vi "TS DotStar SPI V5 - Switched Style.vi"() -> ()   [LabVIEW 2016]
doc: "ADXL362 SPI Accelerometer\n\nThis example shows how to use the Analog Devices ADXL362 Accelerometer sensor connected to SPI.\n\nThis example expects a USB cable connected from your development PC to the Type B USB Jack (next to the power input) on the roboRIO."
uses:
  <vilib>/Rock Robotics/SystemInterfaces/spilib/spi_bus.ctl
  <vilib>/Rock Robotics/WPI/SPI/WPI_SPIMode.ctl
panel:
  in  "Global Max\nBrightness":u8(slide)=4 max=31 scale=0.0..31.0
  in  "line up":bool
  in  "Number of Lights":u8
  out "ONOFF":bool
  in  "Blink Rate":u32
  in  "Blinky End":u8
  in  "Chip Select Active High (F)":bool
  in  "Mode (3)":T1=enum."Mode 3 (Clk Idle High,Sample on Trailing)"
  in  "Clock Rate (Hz)":dbl=500000.0
  in  "error in":errorcluster
  in  "SPI Bus":T2=enum."SPI On-Board, CS1"
  out "error out":errorcluster
  in  "stop":bool
  # "Set these inputs before running."
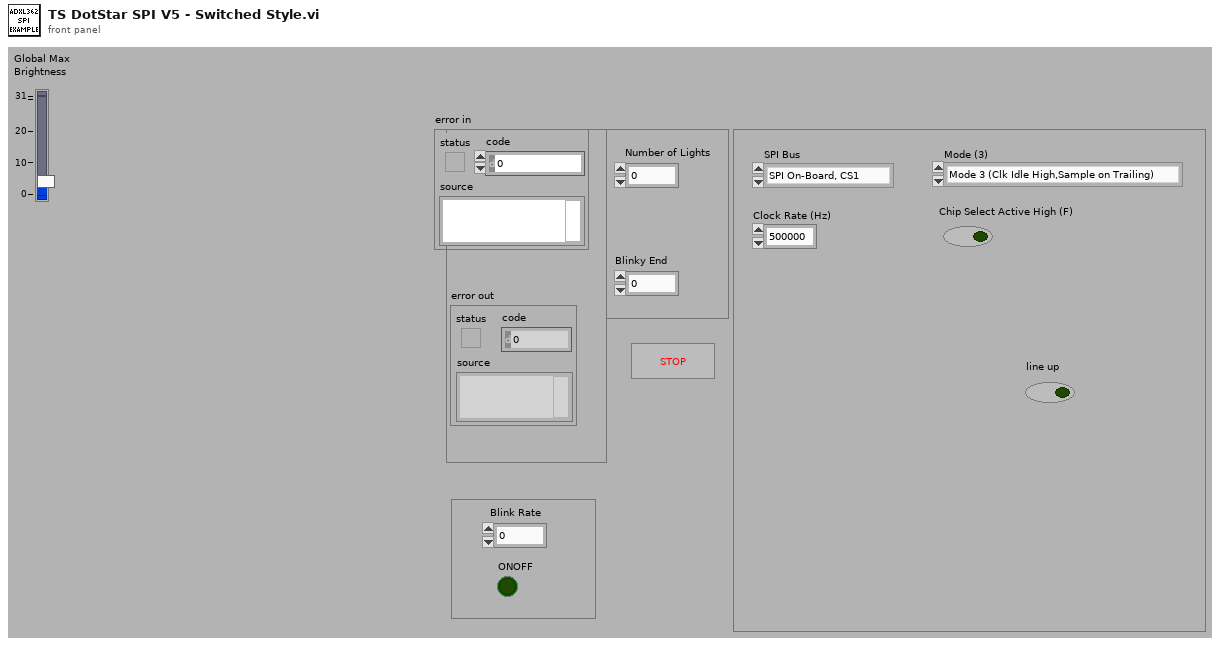
[diagram p1: front panel]
types:
  T1 = typedef "WPI_SPIMode.ctl" = enum16{"Mode 0 (Clk Idle Low,Sample on Leading)", "Mode 1 (Clk Idle Low,Sample on Trailing)", "Mode 2 (Clk Idle High,Sample on Leading)", "Mode 3 (Clk Idle High,Sample on Trailing)"}
  T2 = typedef "spi_bus.ctl" = enum16{"SPI On-Board, CS0", "SPI On-Board, CS1", "SPI On-Board, CS2", "SPI On-Board, CS3", "SPI MXP", "Invalid"}
  T3 = typedef "WPI_SPIDevRef.ctl" = cluster{"DevStatus":errorcluster, "Handle":i32, "SPI Bus":T2}
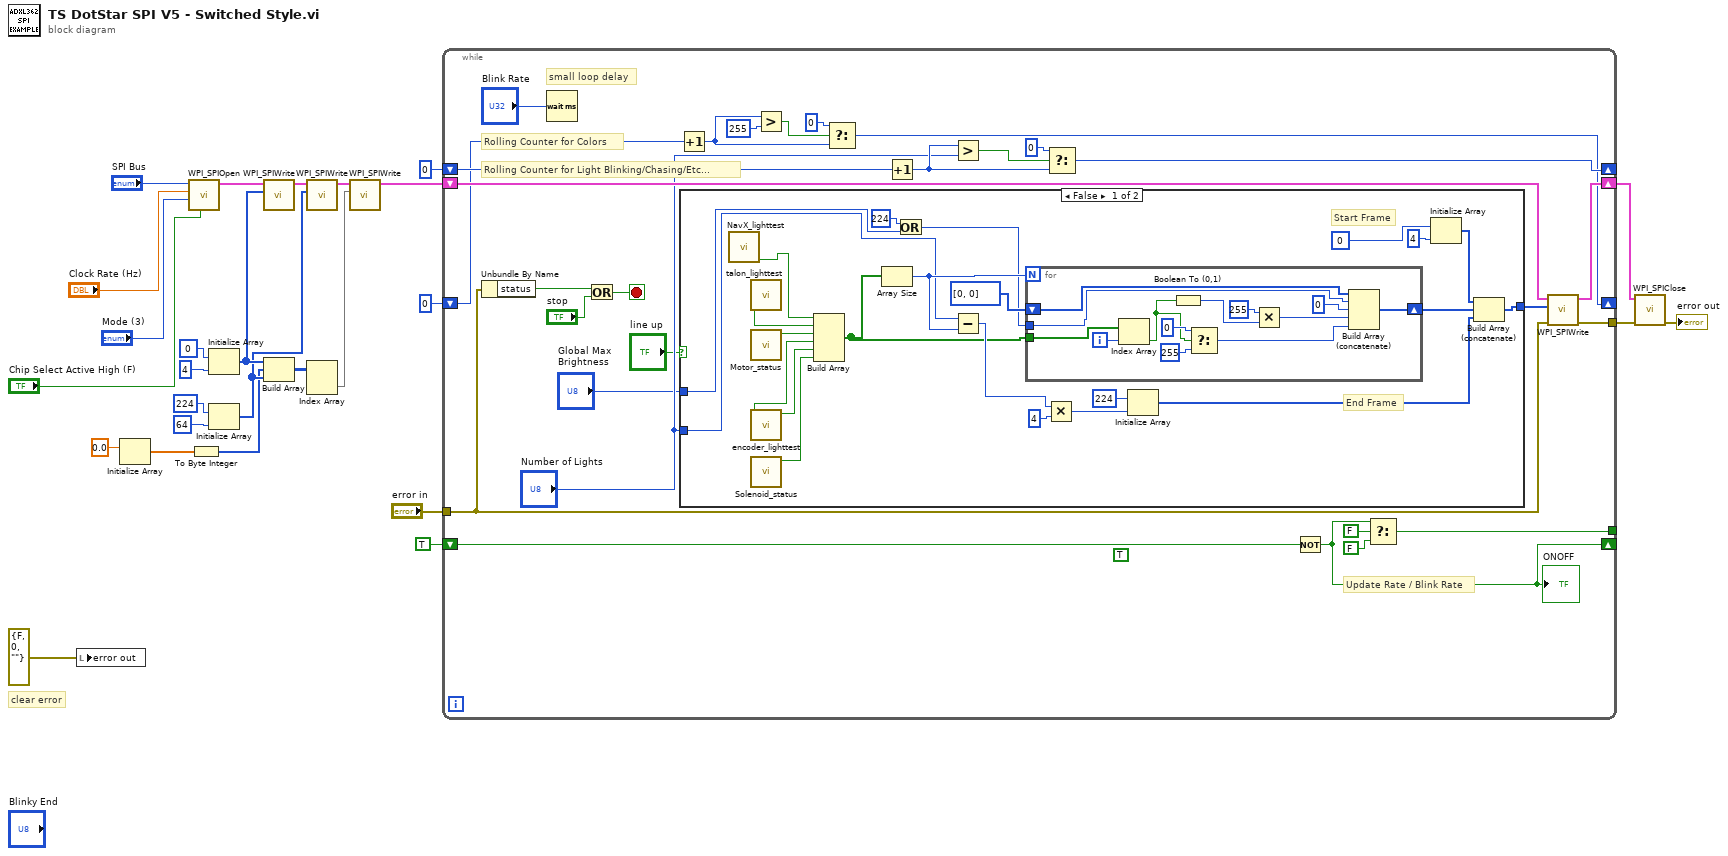
[diagram p0: block diagram]
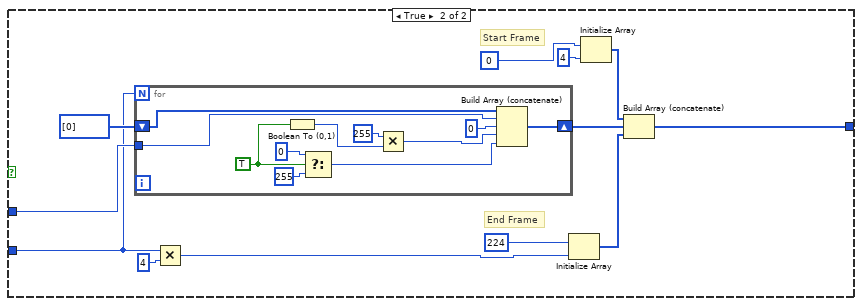
[diagram p2: hidden frame]
diagram:
  # "clear error"
  n1 = local write "error out"(errorcluster {"status"=FALSE, "code"=0, "source"=""} ("error out")) -> ()
  n2 = Initialize Array(0.0 ("element")) -> (w4:dbl[])  [unwired: 1 in]
  n3 = call <vilib>:"WPI_SPIOpen.vi"("Chip Select Active High (F)"="Chip Select Active High (F)", "Mode (3)"="Mode (3)", "Clock Rate (Hz)"="Clock Rate (Hz)", "SPI Bus"="SPI Bus") -> ("SPIDevRef"=w17:T3)  [unwired: 6 in, 1 out]
  n4 = To Byte Integer(number=w4) -> (8bit integer=w3:i8[])
  n5 = Initialize Array(u8 0 ("Data To Send"), u8 4 ("dimension size")) -> (w9:u8[])
  n6 = Initialize Array(u8 224 ("Data To Send"), u8 64 ("dimension size")) -> (w8:u8[])
  n7 = call <vilib>:"WPI_SPIWrite.vi"("Data To Send"=w9, "SPIDevRef"=w17) -> ("SPIDevRef"=w13:T3)  [unwired: 7 in, 2 out]
  n8 = Build Array(w9, w3, w8) -> (w2:u8[][])
  n9 = call <vilib>:"WPI_SPIWrite.vi"("Data To Send"=w8, "SPIDevRef"=w13) -> ("SPIDevRef"=w6:T3)  [unwired: 7 in, 2 out]
  n10 = Index Array(array=w2) -> (element=w1:u8[])  [unwired: 2 in]
  n11 = call <vilib>:"WPI_SPIWrite.vi"("Data To Send"=w1, "SPIDevRef"=w6) -> ("SPIDevRef"=w7:T3)  [unwired: 7 in, 2 out]
  n12 = while {
    shift-right: [w54] -> w24
    shift-left: w7 -> [w52]
    tunnel: "error in" -> [w50]
    tunnel: [w53] -> w14
    tunnel: [w45] -> _
    shift-right: [w43] -> _
    shift-left: TRUE -> [w44]
    shift-right: [w39] -> _
    shift-left: 0 -> [w38]
    shift-right: [w34] -> _
    shift-left: 0 -> [w32]
    stop <- w49 stop-if-true
    (unwired) TRUE
    # "Update Rate / Blink Rate"
    # "Rolling Counter for Light Blinking/Chasing/Etc..."
    # "Rolling Counter for Colors"
    # "small loop delay"
    n13 = Unbundle By Name(w50) -> ("status"=w51:bool)
    n14 = Wait (ms)(milliseconds to wait="Blink Rate") -> ()  [unwired: 1 out]
    n15 = Or(x=w51, y="stop") -> (x .or. y?=w49:bool)
    n16 = Increment(x=w32) -> (x+1=w35:u8)
    n17 = case shown="False" "line up" {
      tunnel: "Number of Lights" -> [w59 w96]
      tunnel: [w58 w93] -> w29
      tunnel: "Global Max\nBrightness" -> [w57 w103]
      frame False {
        # "End Frame"
        # "Start Frame"
        n18 = call "NavX_lighttest.vi"() -> ("NavX_test"=w56:bool)  [unwired: 11 in]
        n19 = call "talon_lighttest.vi"() -> ("Boolean"=w61:bool)  [unwired: 11 in]
        n20 = call "Motor_status.vi"() -> ("Motor Status"=w62:bool)  [unwired: 11 in]
        n21 = call "encoder_lighttest.vi"() -> ("R Encoder"=w64:bool, "L Encoder"=w63:bool)  [unwired: 10 in]
        n22 = call "Solenoid_status.vi"() -> ("Solenoid Status"=w65:bool)  [unwired: 11 in]
        n23 = Build Array(w56, w61, w62, w63, w64, w65) -> (w67:bool[])
        n24 = Array Size(array=w67) -> (size(s)=w71:i32)
        n25 = Or(x=u8 224, y=w57) -> (x .or. y?=w66:u8)
        n26 = Subtract(x=w59, y=w71) -> (x-y=w72:i32)
        n27 = for {
          N: w71 -> [_]
          tunnel: w66 -> [w87]
          tunnel: w67 -> [w80]
          shift-right: [w83] -> w77
          shift-left: i16[] [0, 0] -> [w82]
          i -> [w81]
          n28 = Index Array(array=w80, index=w81) -> (element=w79:bool)
          n29 = Boolean To (0,1)(Boolean=w79) -> (0, 1=w90:i16)
          n30 = Select(t=u8 0, s=w79, f=u8 255) -> (s? t:f=w84:u8)
          n31 = Multiply(x=u8 255, y=w90) -> (x*y=w85:i16)
          n32 = Build Array (concatenate)(w82, w87, u8 0 ("element"), w85, w84) -> (w83:i16[])
        }
        n33 = Multiply(x=w72, y=4) -> (x*y=w74:i32)
        n34 = Initialize Array(u8 224 ("Data To Send"), w74) -> (w76:u8[])
        n35 = Initialize Array(u8 0 ("Data To Send"), u8 4 ("dimension size")) -> (w75:u8[])
        n36 = Build Array (concatenate)(w75, w77, w76) -> (w58:i16[])
      }
      frame True {
        # "End Frame"
        # "Start Frame"
        n37 = for {
          N: w96 -> [_]
          tunnel: w103 -> [w109]
          shift-right: [w105] -> w97
          shift-left: i16[] [0] -> [w104]
          w110 = TRUE
          n38 = Boolean To (0,1)(Boolean=w110) -> (0, 1=w113:i16)
          n39 = Select(t=u8 0, s=w110, f=u8 255) -> (s? t:f=w106:u8)
          n40 = Multiply(x=u8 255, y=w113) -> (x*y=w107:i16)
          n41 = Build Array (concatenate)(w104, w109, u8 0 ("element"), w107, w106) -> (w105:i16[])
        }
        n42 = Multiply(x=w96, y=4) -> (x*y=w98:i32)
        n43 = Initialize Array(u8 224 ("Data To Send"), w98) -> (w95:u8[])
        n44 = Initialize Array(u8 0 ("Data To Send"), u8 4 ("dimension size")) -> (w94:u8[])
        n45 = Build Array (concatenate)(w94, w97, w95) -> (w93:i16[])
      }
    }
    n46 = Greater?(x=w35, y=255) -> (0:w36:bool)
    n47 = Select(t=0, s=w36, f=w35) -> (s? t:f=w34:i32)
    n48 = Increment(x=w38) -> (x+1=w40:u8)
    n49 = Greater?(x=w40, y="Number of Lights") -> (0:w41:bool)
    n50 = Select(t=0, s=w41, f=w40) -> (s? t:f=w39:i32)
    n51 = Not(x=w44) -> (.not. x?=w43:bool)
    "ONOFF" <- w43
    n52 = Select(t=w43, s=FALSE, f=FALSE) -> (s? t:f=w45:bool)
    n53 = call <vilib>:"WPI_SPIWrite.vi"("error in (no error)"=w50, "Data To Send"=w29, "SPIDevRef"=w52) -> ("error out"=w53:errorcluster, "SPIDevRef"=w54:T3)  [unwired: 6 in, 1 out]
  }
  n54 = call <vilib>:"WPI_SPIClose.vi"("error in (no error)"=w14, "SPIDevRef"=w24) -> ("error out"=→"error out":errorcluster)  [unwired: 9 in]
